vi "Voltage_To_U.vi"(7 "Voltages In (Volts)":dbl[](array[numeric]), 13 "Mirror Max Voltage (Volts)":dbl=300.0 format="%#_13g") -> (8 "Pixel Value (-1 to 1)":dbl[](array[numeric]))   [LabVIEW 2014]
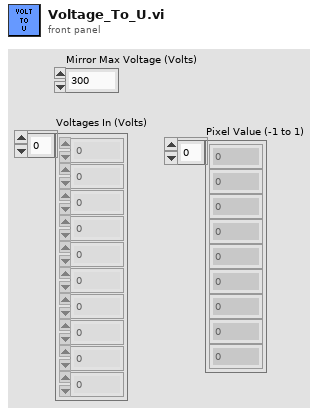
[diagram p1: front panel]
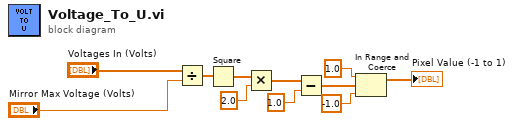
[diagram p0: block diagram]
diagram:
  n1 = Divide(x="Voltages In (Volts)", y="Mirror Max Voltage (Volts)") -> (x/y=w9:dbl[])
  n2 = Square(x=w9) -> (x^2=w8:dbl[])
  n3 = Multiply(x=w8, y=2.0) -> (x*y=w6:dbl[])
  n4 = Subtract(x=w6, y=1.0) -> (x-y=w4:dbl[])
  n5 = In Range and Coerce(upper limit=1.0, x=w4, lower limit=-1.0) -> (coerced(x)=→"Pixel Value (-1 to 1)":dbl[])  [unwired: 1 out]
